vi "Set_offset.vi"(1 "OFFSET UNIT":string, 2 "OFFSET VALUE in":dbl) -> (0 "OFFSET VALUE out":dbl)   [LabVIEW 2019]
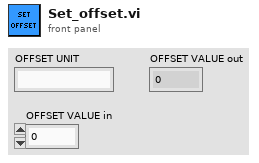
[diagram p1: front panel]
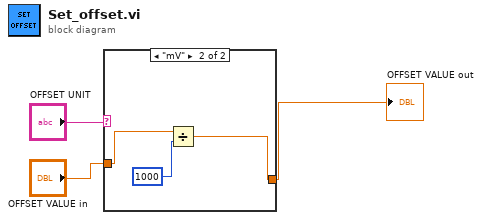
[diagram p0: block diagram]
diagram:
  n1 = case shown="\"mV\"" "OFFSET UNIT" {
    tunnel: "OFFSET VALUE in" -> [w4 w7]
    tunnel: [w4 w5] -> w3
    frame "V", Default {
    }
    frame "mV" {
      n2 = Divide(x=w7, y=1000) -> (x/y=w5:dbl)
    }
  }
  "OFFSET VALUE out" <- w3
